vi "Append Control Value.vi"(9 "Variant Data":variant, 10 "Name":string, 11 "Control Values":cluster{"Name":string, "Variant Data":variant}[](array[cluster])) -> (3 "Control Values":cluster{"Name":string, "Variant Data":variant}[](array[cluster]))   [LabVIEW 2020, in "Responsive Mock.lvclass"]
uses:
  Responsive Mock.lvclass
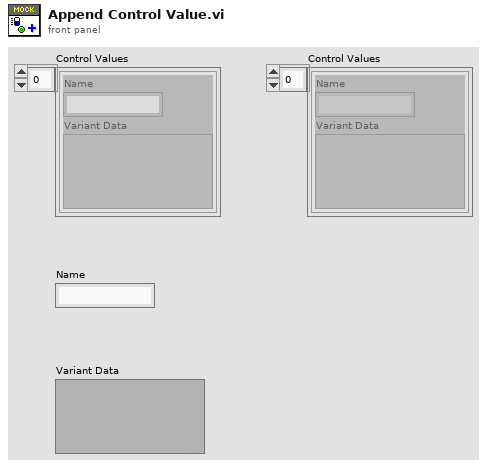
[diagram p1: front panel]
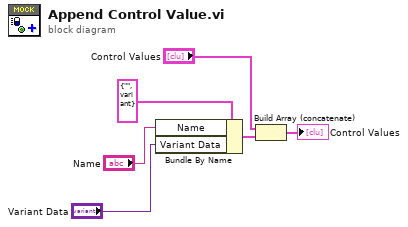
[diagram p0: block diagram]
diagram:
  n1 = Bundle By Name(cluster=cluster{"Name":string, "Variant Data":variant} {"Name"="", "Variant Data"=variant} ("element"), "Name"="Name", "Variant Data"="Variant Data") -> (w4:cluster{"Name":string, "Variant Data":variant})
  n2 = Build Array (concatenate)("Control Values", w4) -> (→"Control Values":cluster{"Name":string, "Variant Data":variant}[])
